vi "Delete and Replace String Section (SubVI).vi"(9 "Length":i32, 10 "Secondary String In":string, 11 "Function String":string) -> (3 "Secondary String Out":string)   [LabVIEW 2012]
doc: "Replaces a section of a string with the function string."
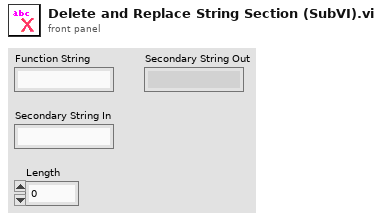
[diagram p1: front panel]
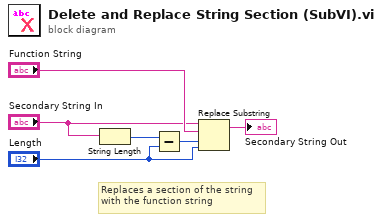
[diagram p0: block diagram]
diagram:
  # "Replaces a section of the string\nwith the function string"
  n1 = String Length(string="Secondary String In") -> (length=w1:i32)
  n2 = Subtract(x=w1, y="Length") -> (x-y=w3:i32)
  n3 = Replace Substring(2:"Length", 3:w3, 4:"Function String", 5:"Secondary String In") -> (1:→"Secondary String Out":string)  [unwired: 1 out]
